vi "Example Caraya CLI.vi"() -> ()   [LabVIEW 2013]
uses:
  <vilib>/Utility/sysdir.llb/System Directory Type.ctl
  <userlib>/_OpenG.lib/file/file.llb/File Exists - Scalar__ogtk.vi
panel:
  out "Command Line string":string
  in  "Output file":path
  out "error out":errorcluster
  in  "LabVIEW EXE path":path=path "C:/Program Files (x86)/National Instruments/LabVIEW 2014/LabVIEW.exe"
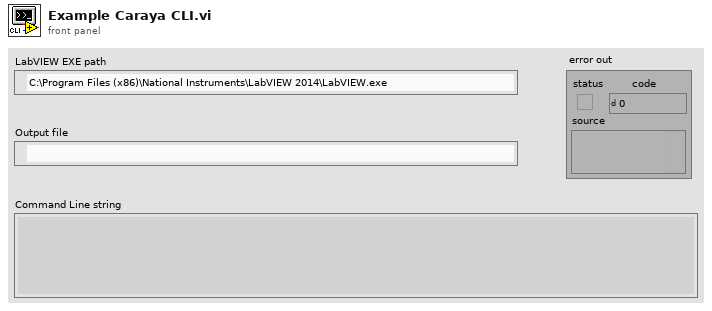
[diagram p1: front panel]
types:
  T1 = typedef "System Directory Type.ctl" = i32
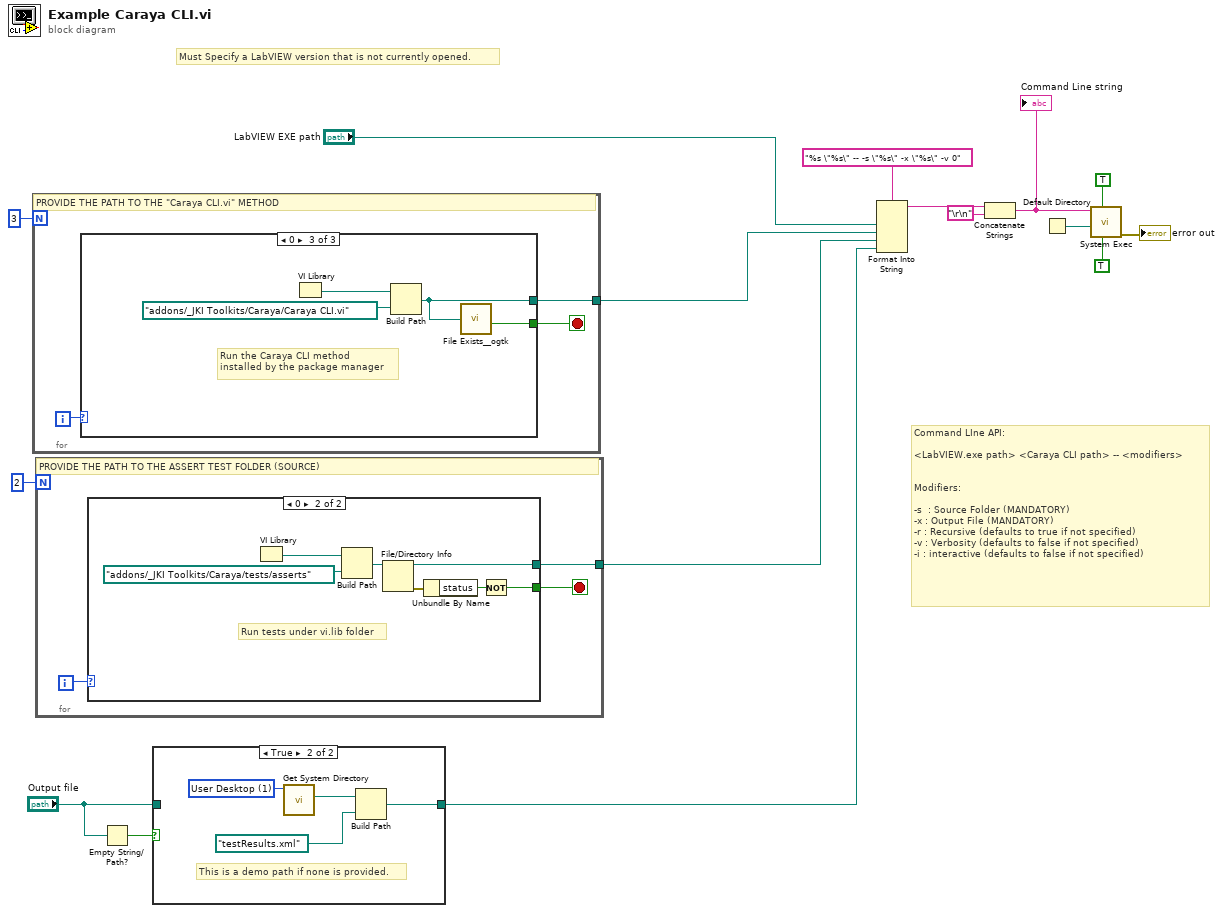
[diagram p0: block diagram]
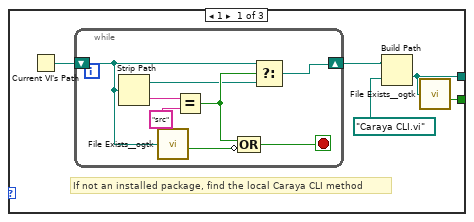
[diagram p3: hidden frame]
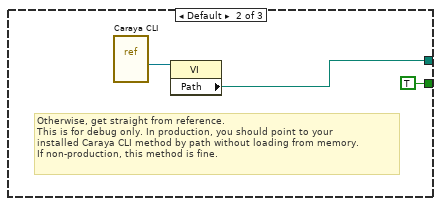
[diagram p4: hidden frame]
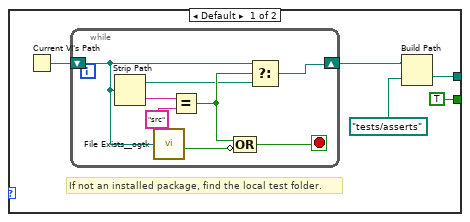
[diagram p5: hidden frame]
diagram:
  # "Must Specify a LabVIEW version that is not currently opened."
  # "Command LIne API:\n\n<LabVIEW.exe path> <Caraya CLI path> -- <modifiers>\n\n\nModifiers: \n\n-s  : Source Folder (MANDATORY)\n-x : Output File (MANDATORY)\n-r : Recursive (defaults to true if not specified)\n-v : Verbosity (defaults to false if not specified)\n-i : interactive (defaults to false if not specified)"
  n1 = for {
    N: 3 -> [_]
    tunnel: [w18] -> w3
    i -> [w17]
    stop <- w19 stop-if-true
    # "PROVIDE THE PATH TO THE \"Caraya CLI.vi\" METHOD"
    n2 = case shown="0" w17 {
      tunnel: [w20 TRUE ("exists") w37] -> w19
      tunnel: [w21 w34 w36] -> w18
      frame 1 {
        # "If not an installed package, find the local Caraya CLI method"
        n3 = Current VI's Path() -> (path=w24:path)
        n4 = while {
          shift-right: [w26] -> w23
          shift-left: w24 -> [w27]
          stop <- w29 stop-if-true
          n5 = Strip Path(path=w27) -> (stripped path=w25:path, name=w32:string)
          n6 = call-poly <userlib>:"File Exists__ogtk.vi"("file path"=w27) -> ("exists"=w30:bool)  [unwired: 6 in, 1 out]
          n7 = Equal?(x=w32, y="src") -> (x = y?=w28:bool)
          n8 = Compound Arithmetic op=OR(w28, invert w30) -> (w29:bool)
          n9 = Select(t=w27, s=w28, f=w25) -> (s? t:f=w26:path)
        }
        n10 = Build Path(base path=w23, name or relative path=path "Caraya CLI.vi") -> (appended path=w21:path)
        n11 = call-poly <userlib>:"File Exists__ogtk.vi"("file path"=w21) -> ("exists"=w20:bool)  [unwired: 6 in, 1 out]
      }
      frame Default {
        # "Otherwise, get straight from reference.\nThis is for debug only. In production, you should point to your\ninstalled Caraya CLI method by path without loading from memory. \nIf non-production, this method is fine."
        n12 = vi-ref "Caraya CLI.vi"() -> (w35:refnum<vi>)
        n13 = property class="VI"(reference=w35) -> ("Path"=w34:path)  [unwired: 1 in, 2 out]
      }
      frame 0 {
        # "Run the Caraya CLI method\ninstalled by the package manager"
        n14 = VI Library() -> (path=w39:path)
        n15 = Build Path(base path=w39, name or relative path=path "addons/_JKI Toolkits/Caraya/Caraya CLI.vi") -> (appended path=w36:path)
        n16 = call-poly <userlib>:"File Exists__ogtk.vi"("file path"=w36) -> ("exists"=w37:bool)  [unwired: 6 in, 1 out]
      }
    }
  }
  n17 = for {
    N: 2 -> [_]
    tunnel: [w41] -> w6
    i -> [w40]
    stop <- w42 stop-if-true
    # "PROVIDE THE PATH TO THE ASSERT TEST FOLDER (SOURCE)"
    n18 = case shown="0" w40 {
      tunnel: [TRUE w57] -> w42
      tunnel: [w46 w56] -> w41
      frame Default {
        # "If not an installed package, find the local test folder."
        n19 = Current VI's Path() -> (path=w47:path)
        n20 = while {
          shift-right: [w49] -> w45
          shift-left: w47 -> [w50]
          stop <- w52 stop-if-true
          n21 = Strip Path(path=w50) -> (stripped path=w48:path, name=w55:string)
          n22 = call-poly <userlib>:"File Exists__ogtk.vi"("file path"=w50) -> ("exists"=w53:bool)  [unwired: 6 in, 1 out]
          n23 = Equal?(x=w55, y="src") -> (x = y?=w51:bool)
          n24 = Compound Arithmetic op=OR(w51, invert w53) -> (w52:bool)
          n25 = Select(t=w50, s=w51, f=w48) -> (s? t:f=w49:path)
        }
        n26 = Build Path(base path=w45, name or relative path=path "tests/asserts") -> (appended path=w46:path)
      }
      frame 0 {
        # "Run tests under vi.lib folder"
        n27 = VI Library() -> (path=w62:path)
        n28 = Build Path(base path=w62, name or relative path=path "addons/_JKI Toolkits/Caraya/tests/asserts") -> (appended path=w58:path)
        n29 = File/Directory Info(path=w58) -> (path out=w56:path, error out=w60:errorcluster)  [unwired: 1 in, 5 out]
        n30 = Unbundle By Name(w60) -> ("status"=w59:bool)
        n31 = Not(x=w59) -> (.not. x?=w57:bool)
      }
    }
  }
  n32 = Empty String/Path?(string/path="Output file") -> (empty?=w2:bool)
  n33 = case shown="True" w2 {
    tunnel: [w63 w64] -> w5
    tunnel: "Output file" -> [w63 _]
    frame False {
    }
    frame True {
      w67 = T1 1 items=["User Home"=0, "User Desktop"=1, "User Documents"=2, "User Application Data"=3, "User Preferences"=4, "User Temporary"=5, "Public Documents"=6, "Public Application Data"=7, "Public Preferences"=8, "Public Cache"=13, "System Core Libraries"=9, "System Installed Libraries"=10, "Application Files"=11, "Boot Volume Root"=12] ("system directory type")
      # "This is a demo path if none is provided."
      n34 = call <vilib>:"Get System Directory.vi"("system directory type"=w67) -> ("system directory"=w66:path)  [unwired: 10 in]
      n35 = Build Path(base path=w66, name or relative path=path "testResults.xml") -> (appended path=w64:path)
    }
  }
  n36 = Format Into String(format string="%s \"%s\" -- -s \"%s\" -x \"%s\" -v 0", "LabVIEW EXE path", w3, w6, w5) -> (resulting string=w10:string)  [unwired: 2 in, 1 out]
  n37 = Concatenate Strings(w10, "\r\n") -> (w12:string)
  "Command Line string" <- w12
  n38 = Default Directory() -> (w9:path)
  n39 = call <vilib>:"System Exec.vi"("run minimized? (F)"=TRUE, "wait until completion? (T)"=TRUE, "working directory"=w9, "command line"=w12) -> ("error out"=→"error out":errorcluster)  [unwired: 4 in, 3 out]
